vi "InvokeGlobalEvent.vi"(8 "error in (no error)":errorcluster, 9 "Invoke?":bool=TRUE, 10 "Data":variant, 11 "name":string) -> (0 "error out":errorcluster)   [LabVIEW 2017]
uses:
  Globals/globals.vi
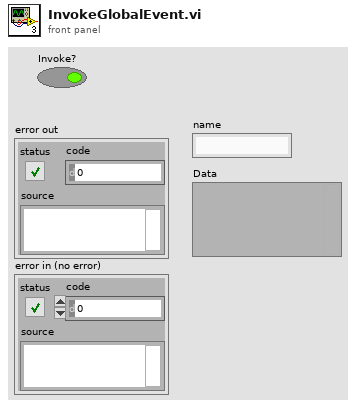
[diagram p1: front panel]
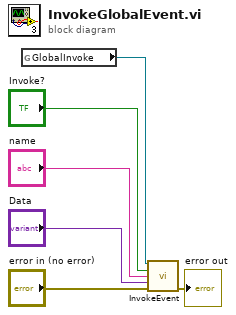
[diagram p0: block diagram]
diagram:
  n1 = global read "globals.vi" "GlobalInvoke"() -> (w3:refnum<user-event>)
  n2 = call "InvokeEvent.vi"("User Event in"=w3, "Invoke?"="Invoke?", "name"="name", "Data"="Data", "error in (no error)"="error in (no error)") -> ("error out"=→"error out":errorcluster)  [unwired: 9 in, 1 out]
